vi "Power Meter.vi"(8 "error in (no error)":errorcluster, 11 "Power Meter in":refnum<class "Power Meter.lvclass">) -> (0 "error out":errorcluster, 3 "Power Meter out":refnum<class "Power Meter.lvclass">)   [LabVIEW 2012, in "Power Meter.lvclass"]
uses:
  Power Meter.lvclass
  Utility Classes/Readable/Channel Names.ctl
  Power Meter.lvclass/Power Meter.ctl
  Global/GPIB Numbers.vi
  Utility Classes/Readable/Readable.lvclass
panel:
  out "Status":string
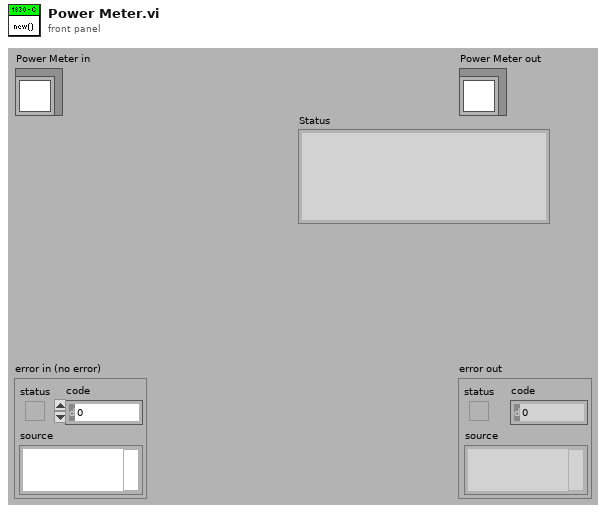
[diagram p1: front panel]
types:
  T1 = typedef "Readable.lvclass/Channel Names.ctl" = string[]
  T2 = typedef "GPIB Type Def.ctl" = cluster{"Name":string, "bus":dbl, "GPIB":dbl, "GPIB as string":string, "byte":i32, "VISA Resource Name":refnum<visa-resource-name>}
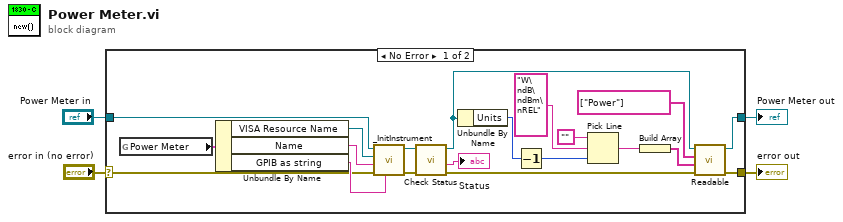
[diagram p0: block diagram]
diagram:
  n1 = case shown="No Error" "error in (no error)" {
    selector: "error in (no error)" -> [w16 w26]
    tunnel: [w13 w26] -> w3
    tunnel: [w15 w25] -> w1
    tunnel: "Power Meter in" -> [w21 w25]
    frame No Error {
      n2 = global read "GPIB Numbers.vi" "Power Meter"() -> (w24:T2)
      n3 = Unbundle By Name(w24) -> ("VISA Resource Name"=w20:refnum<visa-resource-name>, "Name"=w17:string, "GPIB as string"=w19:string)
      n4 = call-dynamic "_InitInstrument.vi"("GPIB as string"=w19, "error in (no error)"=w16, "Name"=w17, "VISA Resource Name"=w20, "Instrument in"=w21) -> ("error out"=w18:errorcluster, "Instrument out"=w23:refnum<class "Power Meter.lvclass">)  [unwired: 1 in, 4 out]
      n5 = call-dynamic "Check Status.vi"("error in (no error)"=w18, "Power Meter in"=w23) -> ("error out"=w14:errorcluster, "Status"=→"Status":string, "Power Meter out"=w11:refnum<class "Power Meter.lvclass">)  [unwired: 6 in, 1 out]
      n6 = Unbundle By Name(w11) -> ("Units"=w10:u16)
      n7 = Decrement(x=w10) -> (x-1=w7:u16)
      n8 = Pick Line(string ("")="", multi-line string="W\ndB\ndBm\nREL", line index=w7) -> (output string=w6:string)
      n9 = Build Array(w6) -> (w5:string[])
      n10 = call "Readable.vi"("error in (no error)"=w14, "Channel Units"=w5, "Channel Names"=T1 ["Power"], "Readable in"=w11) -> ("error out"=w13:errorcluster, "Readable out"=w15:refnum<class "Power Meter.lvclass">)  [unwired: 6 in]
    }
    frame Error {
    }
  }
  "error out" <- w3
  "Power Meter out" <- w1
